vi "Arm Encoder Control.vi"(8 "Channels":string[](array[string]), 10 "Reset":bool, 11 "Enum":T1) -> (2 "Distance (In)":dbl, 3 "Rate":dbl)   [LabVIEW 2014]
uses:
  SRE Enum.ctl
  <vilib>/Rock Robotics/WPI/Counter/WPI_CounterDigitalInputToDigitalSource.vi
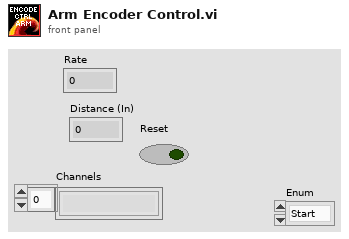
[diagram p1: front panel]
types:
  T1 = typedef "SRE Enum.ctl" = enum16{"Start", "Run", "End"}
  T2 = typedef "WPI_DigitalInputDevRef.ctl" = cluster{"DevStatus":errorcluster, "DIO Channel":T3, "Controller":T4}
  T3 = typedef "FPGA_DIOChannel.ctl" = enum8{"DIO 0", "DIO 1", "DIO 2", "DIO 3", "DIO 4", "DIO 5", "DIO 6", "DIO 7", "DIO 8", "DIO 9", "DIO MXP 0", "DIO MXP 1", "DIO MXP 2", "DIO MXP 3", "DIO MXP 4", "DIO MXP 5", "DIO MXP 6", "DIO MXP 7", "DIO MXP 8", "DIO MXP 9", "DIO MXP 10", "DIO MXP 11", "DIO MXP 12", "DIO MXP 13", "DIO MXP 14", "DIO MXP 15", "Invalid"}
  T4 = typedef "FPGA_TypedefDigitalModule.ctl" = enum16{"Controller 1"}
  T5 = typedef "FPGA_CounterEncoderSourceConvertionLVSourceType.ctl" = cluster{"DevStatus":errorcluster, "AnalogTriggerMode?":bool, "DigitalMode":cluster{"Controller":T4, "DIO Channel":T6}, "AnalogTriggerMode":cluster{"AnalogTriggerIndex":T7, "OutputType":T8}}
  T6 = typedef "FPGA_DIODigitalSourceChannel.ctl" = enum8{"DIO 0", "DIO 1", "DIO 2", "DIO 3", "DIO 4", "DIO 5", "DIO 6", "DIO 7", "DIO 8", "DIO 9", "DIO MXP 0", "DIO MXP 1", "DIO MXP 2", "DIO MXP 3", "DIO MXP 4", "DIO MXP 5", "DIO MXP 6", "DIO MXP 7", "DIO MXP 8", "DIO MXP 9", "DIO MXP 10", "DIO MXP 11", "DIO MXP 12", "DIO MXP 13", "DIO MXP 14", "DIO MXP 15", "Disabled"}
  T7 = typedef "FPGA_AnalogTriggerIndex.ctl" = enum8{"Trig 0", "Trig 1", "Trig 2", "Trig 3", "Trig 4", "Trig 5", "Trig 6", "Trig 7", "Invalid"}
  T8 = typedef "FPGA_AnalogTriggerOutType.ctl" = enum16{"InWindow", "TriggerState", "Rising", "Falling"}
  T9 = typedef "WPI_EncoderDevRef.ctl" = cluster{"DevStatus":errorcluster, "EncoderIndex":T10, "CounterIndex":T11, "DistancePerCount":dbl, "Decoding Type":T12}
  T10 = typedef "FPGA_EncoderIdx.ctl" = enum8{"Enc 0", "Enc 1", "Enc 2", "Enc 3", "Enc 4", "Enc 5", "Enc 6", "Enc 7", "Invalid"}
  T11 = typedef "FPGA_CounterCtrSystemIndex.ctl" = enum8{"Ctr 0", "Ctr 1", "Ctr 2", "Ctr 3", "Ctr 4", "Ctr 5", "Ctr 6", "Ctr 7", "Invalid"}
  T12 = typedef "WPI_EncoderType.ctl" = enum16{"1x", "2x", "4x"}
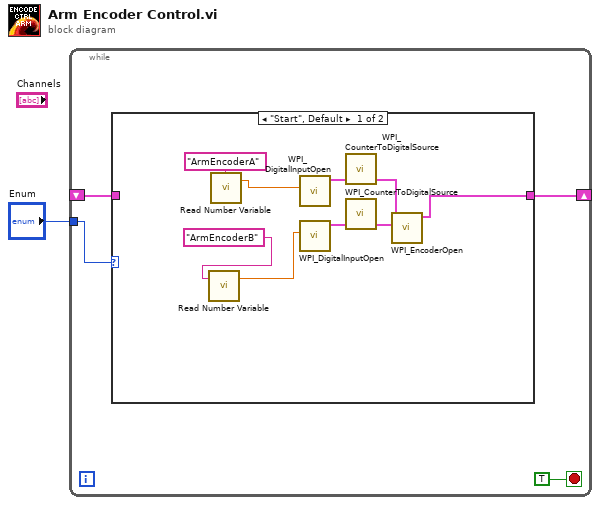
[diagram p0: block diagram]
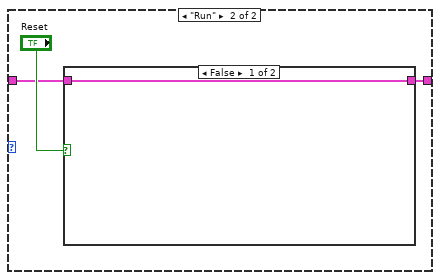
[diagram p2: hidden frame]
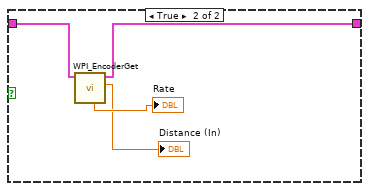
[diagram p3: hidden frame]
diagram:
  n1 = while {
    tunnel: "Enum" -> [w5]
    shift-right: [w4] -> _
    shift-left: _ -> [w3]
    stop <- TRUE stop-if-true
    n2 = case shown="\"Start\", Default" w5 {
      tunnel: [w10 w16] -> w4
      tunnel: w3 -> [_ w15]
      frame "Start", Default {
        n3 = call "Read Number Variable.vi"("Name"="ArmEncoderB") -> ("number"=w6:dbl)  [unwired: 1 in, 1 out]
        n4 = call "Read Number Variable.vi"("Name"="ArmEncoderA") -> ("number"=w8:dbl)  [unwired: 1 in, 1 out]
        n5 = call <vilib>:"WPI_DigitalInputOpen.vi"("DIO Channel"=w8) -> ("DigitalInputDevRef"=w12:T2)  [unwired: 2 in, 8 out]
        n6 = call <vilib>:"WPI_DigitalInputOpen.vi"("DIO Channel"=w6) -> ("DigitalInputDevRef"=w13:T2)  [unwired: 2 in, 8 out]
        n7 = call-poly <vilib>:"WPI_CounterToDigitalSource.vi"("DigitalInputDevRef"=w12) -> ("Digital Source"=w11:T5)  [unwired: 6 out]
        n8 = call-poly <vilib>:"WPI_CounterToDigitalSource.vi"("DigitalInputDevRef"=w13) -> ("Digital Source"=w14:T5)  [unwired: 6 out]
        n9 = call <vilib>:"WPI_EncoderOpen.vi"("BSource"=w14, "ASource"=w11) -> ("EncoderDevRef"=w10:T9)  [unwired: 6 in, 3 out]
      }
      frame "Run" {
        n10 = case shown="False" "Reset" {
          tunnel: [w18 w22] -> w16
          tunnel: w15 -> [w18 w21]
          frame False {
          }
          frame True {
            n11 = call <vilib>:"WPI_EncoderGet.vi"("EncoderDevRef"=w21) -> ("Distance"=→"Distance (In)":dbl, "EncoderDevRef"=w22:T9, "Rate"=→"Rate":dbl)  [unwired: 5 in, 3 out]
          }
        }
      }
    }
  }
